vi "XML Write.vi"(7 "XML File Path Write":path=path "c:/config.xml", 8 "Error In":errorcluster, 11 "FOFB Parameters":T1) -> (0 "Error Out":errorcluster, 3 "XML File Path Out":path)   [LabVIEW 2011, in "XML VIs.lvlib"]
uses:
  XML VIs.lvlib
  Types Definitions/Type FOFB Parameters.ctl
  Types Definitions/Type Network Configuration.ctl
  Types Definitions/Type FA Configuration.ctl
  Types Definitions/Type Acquisition Network Configuration.ctl
  Types Definitions/Type Actuation Network Configuration.ctl
  Third Party/GXML/GXML.lvlib
  Type Definitions.lvlib
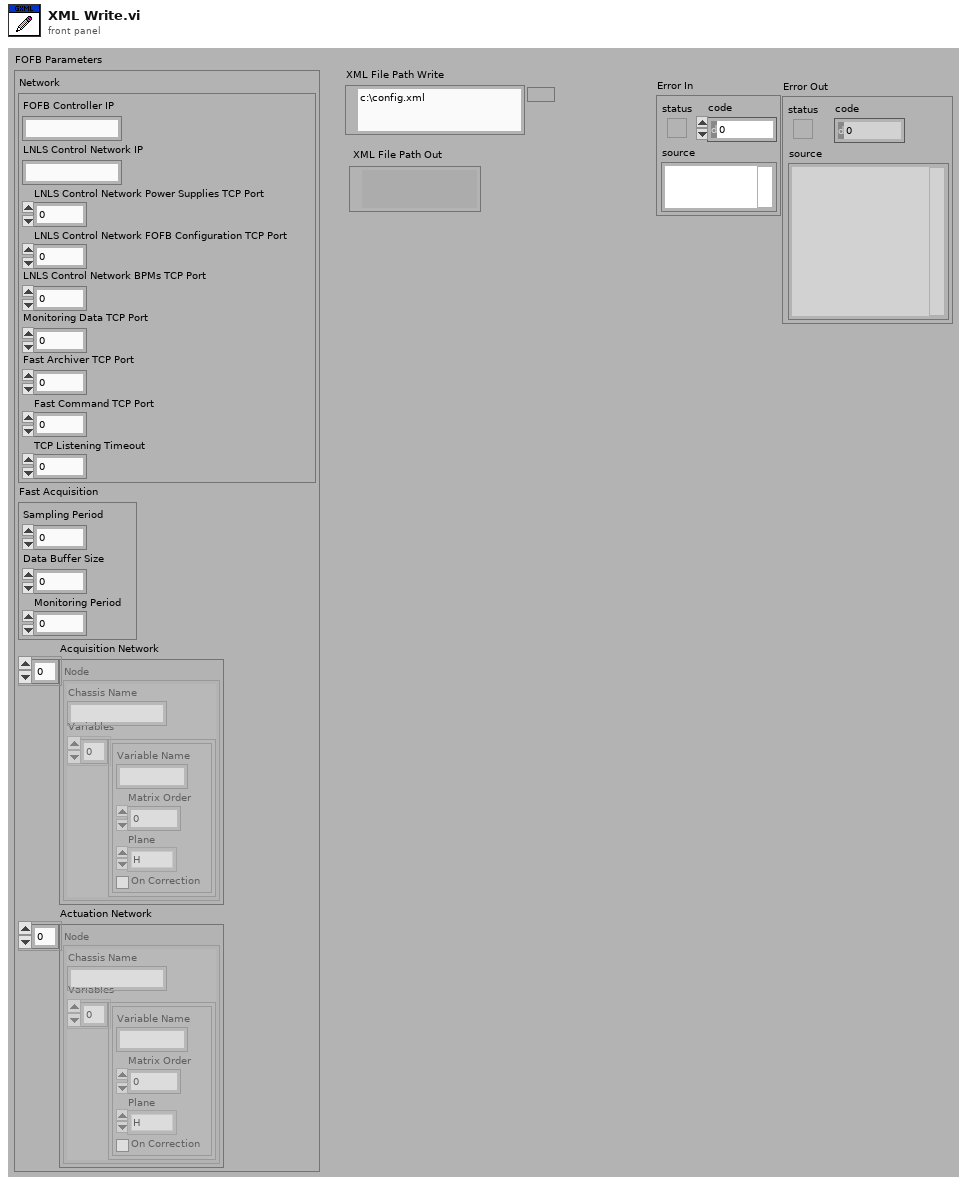
[diagram p1: front panel]
types:
  T1 = typedef "Type Definitions.lvlib/Type FOFB Parameters.ctl" = cluster{"Network":T2, "Fast Acquisition":T3, "Acquisition Network":T4, "Actuation Network":T5}
  T2 = typedef "Type Definitions.lvlib/Type Network Configuration.ctl" = cluster{"FOFB Controller IP":string, "LNLS Control Network IP":string, "LNLS Control Network Power Supplies TCP Port":u16, "LNLS Control Network FOFB Configuration TCP Port":u16, "LNLS Control Network BPMs TCP Port":u16, "Monitoring Data TCP Port":u16, "Fast Archiver TCP Port":u16, "Fast Command TCP Port":u16, "TCP Listening Timeout":i32}
  T3 = typedef "Type Definitions.lvlib/Type FA Configuration.ctl" = cluster{"Sampling Period":u32, "Data Buffer Size":u32, "Monitoring Period":u32}
  T4 = typedef "Type Definitions.lvlib/Type Acquisition Network Configuration.ctl" = cluster{"Chassis Name":string, "Variables":cluster{"Variable Name":string, "Matrix Order":u32, "Plane":enum8{"H", "V"}, "On Correction":bool}[]}[]
  T5 = typedef "Type Definitions.lvlib/Type Actuation Network Configuration.ctl" = cluster{"Chassis Name":string, "Variables":cluster{"Variable Name":string, "Matrix Order":u32, "Plane":enum8{"H", "V"}, "On Correction":bool}[]}[]
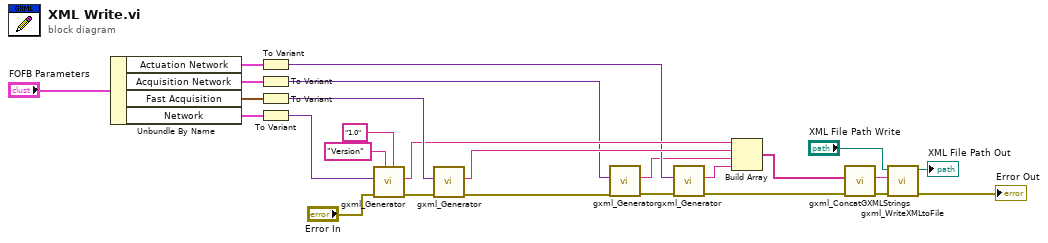
[diagram p0: block diagram]
diagram:
  n1 = Unbundle By Name("FOFB Parameters") -> ("Actuation Network"=w2:T5, "Acquisition Network"=w3:T4, "Fast Acquisition"=w4:T3, "Network"=w5:T2)
  n2 = To Variant(anything=w2) -> (Variant=w9:variant)
  n3 = To Variant(anything=w3) -> (Variant=w10:variant)
  n4 = To Variant(anything=w4) -> (Variant=w15:variant)
  n5 = To Variant(anything=w5) -> (Variant=w16:variant)
  n6 = call "gxml_Generator.vi"("Version String"="1.0", "Version Tag Name"="Version", "error in"="Error In", "Variant"=w16) -> ("error out"=w17:errorcluster, "XML String Out"=w13:string)  [unwired: 6 in]
  n7 = call "gxml_Generator.vi"("error in"=w17, "Variant"=w15) -> ("error out"=w1:errorcluster, "XML String Out"=w14:string)  [unwired: 8 in]
  n8 = call "gxml_Generator.vi"("error in"=w1, "Variant"=w10) -> ("error out"=w12:errorcluster, "XML String Out"=w8:string)  [unwired: 8 in]
  n9 = call "gxml_Generator.vi"("error in"=w12, "Variant"=w9) -> ("error out"=w11:errorcluster, "XML String Out"=w7:string)  [unwired: 8 in]
  n10 = Build Array(w13, w14, w8, w7) -> (w24:string[])
  n11 = call "gxml_ConcatGXMLStrings.vi"("error in"=w11, "GXML Strings"=w24) -> ("error out"=w25:errorcluster, "Concatenated GXML String"=w26:string)  [unwired: 8 in]
  n12 = call "gxml_WriteXMLtoFile.vi"("error in"=w25, "XML Input"=w26, "XML File Path"="XML File Path Write") -> ("error out"=→"Error Out":errorcluster, "XML File Path Out"=→"XML File Path Out":path)  [unwired: 7 in]
